vi "Read Item (SGL).vi"(6 "itemName":string, 8 "error in (no error)":errorcluster, 11 ".NET Refnum in":refnum<k24>) -> (0 "error out":errorcluster, 1 "variant":variant, 2 "Value (SGL/DBL only!)":sgl, 3 ".NET Refnum out":refnum<k24>, 4 "type":T1, 5 "ItemName":string, 7 "Name":string)   [LabVIEW 2024, in "LV_OPC_NET.lvlib"]
uses:
  LV_OPC_NET.lvlib
  <vilib>/Utility/Data Type/Type Definitions/Data Type.ctl
  C:/Users/Andrey/Desktop/LV_OPC-Client-x64/LV_OPC_Test/OPC.NET/OpcNetApi.dll
  OpcNetApi.dll
  System.Xml
  <vilib>/Utility/Data Type/NI_Data Type.lvlib
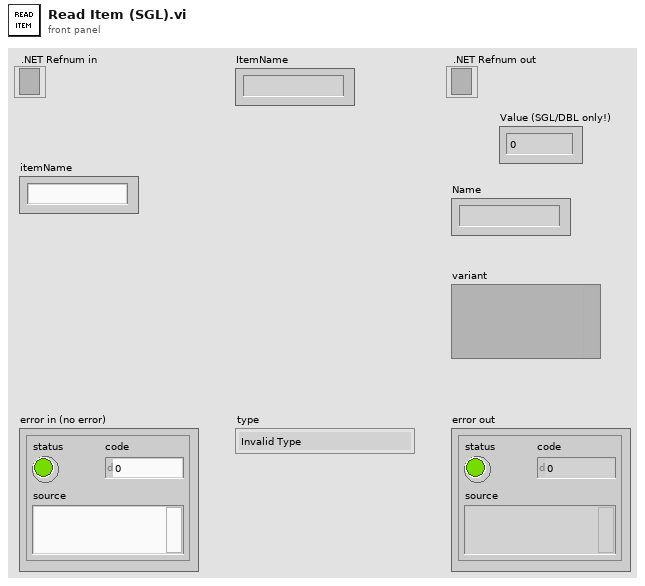
[diagram p1: front panel]
types:
  T1 = typedef "NI_Data Type.lvlib/Data Type.ctl" = enum8{"Invalid Type", "Void", "I8", "I16", "I32", "I64", "U8", "U16", "U32", "U64", "Single Float", "Double Float", "Extended Float", "Single Complex", "Double Complex", "Extended Complex", "Enum U8", "Enum U16", "Enum U32", "Enum U64", "Single Float With Unit", "Double Float With Unit", "Extended Float With Unit", "Single Complex with Unit", "Double Complex with Unit", "Extended Complex with Unit", "Boolean", "String", "Path", "Picture", "Tag", "Array", "Cluster", "Variant", "LV Variant", "Waveform", "Timestamp", "Digital Waveform", "Digital Data", "ExpressData", "Refnum", "External Data", "VI", "Poly VI", "LabVIEW Class Instance", "Fixed Point", "Set Collection", "Map Collection"}
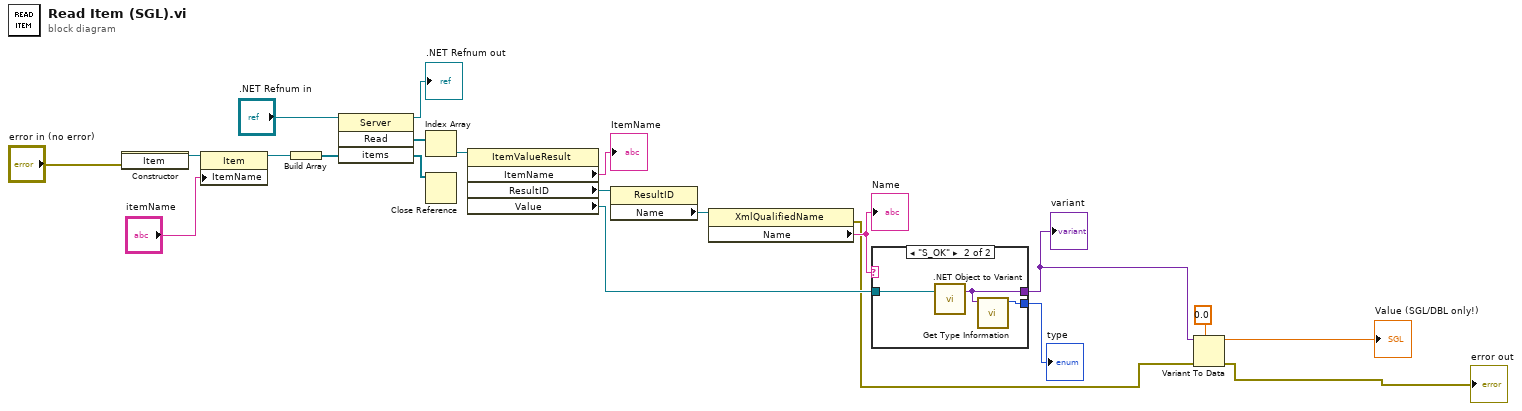
[diagram p0: block diagram]
diagram:
  n1 = constructor class="Item"(error in="error in (no error)") -> (reference out=w9:refnum<k24>)  [unwired: 2 in, 2 out]
  n2 = property class="Item"(reference=w9, "ItemName"="itemName") -> (reference out=w10:refnum<k24>)  [unwired: 1 in, 1 out]
  n3 = Build Array(w10) -> (w11:refnum<k24>[])
  n4 = invoke class="Server" method="Read"(reference=".NET Refnum in", "items"=w11) -> (reference out=→".NET Refnum out":refnum<k24>, "Read"=w17:refnum<k24>[], "items"=w16:refnum<k24>[])  [unwired: 2 in, 1 out]
  n5 = Index Array(array=w17) -> (element=w13:refnum<k24>)  [unwired: 1 in]
  n6 = Close Reference(reference=w16) -> ()  [unwired: 1 in, 1 out]
  n7 = property class="ItemValueResult"(reference=w13) -> ("ItemName"=→"ItemName":string, "ResultID"=w19:refnum<k24>, "Value"=w15:refnum<k24>)  [unwired: 1 in, 2 out]
  n8 = property class="ResultID"(reference=w19) -> ("Name"=w18:refnum<k24>)  [unwired: 1 in, 2 out]
  n9 = property class="XmlQualifiedName"(reference=w18) -> (error out=w3:errorcluster, "Name"=w20:string)  [unwired: 1 in, 1 out]
  "Name" <- w20
  n10 = case shown="\"S_OK\"" w20 {
    tunnel: w15 -> [_ w24]
    tunnel: [_ w23] -> w6
    tunnel: [_ w22] -> w5
    frame Default {
    }
    frame "S_OK" {
      n11 = call <vilib>:".NET Object to Variant.vi"(".NET object"=w24) -> ("variant"=w22:variant)  [unwired: 1 in, 1 out]
      n12 = call <vilib>:"Get Type Information.vi"("variant"=w22) -> ("type"=w23:T1)  [unwired: 6 in, 4 out]
    }
  }
  "variant" <- w5
  "type" <- w6
  n13 = Variant To Data(error in=w3, type=sgl 0.0, Variant=w5) -> (data=→"Value (SGL/DBL only!)":sgl, error out=→"error out":errorcluster)
